vi "NortekCommander.vi"(4 "error in (no error)":errorcluster) -> ()   [LabVIEW 2015]
uses:
  Globals/NortekInstruction.vi
panel:
  out "number":u32
  in  "Stop_Rec":bool
  in  "Start_Rec":bool
  in  "MesureOne":bool
  in  "nom":bool
  out "error out":errorcluster
  out "data out":string
  in  "Date ?":bool
  out "iteration":i32
  in  "Server Closed":string="The server VI closed the connection."
  in  "Stop":bool
  # "Nortek Commander"
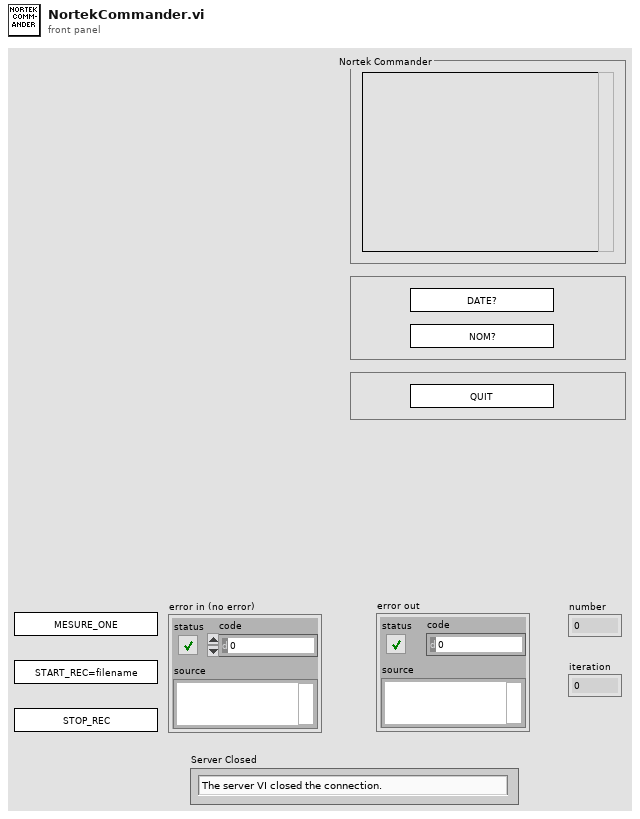
[diagram p1: front panel]
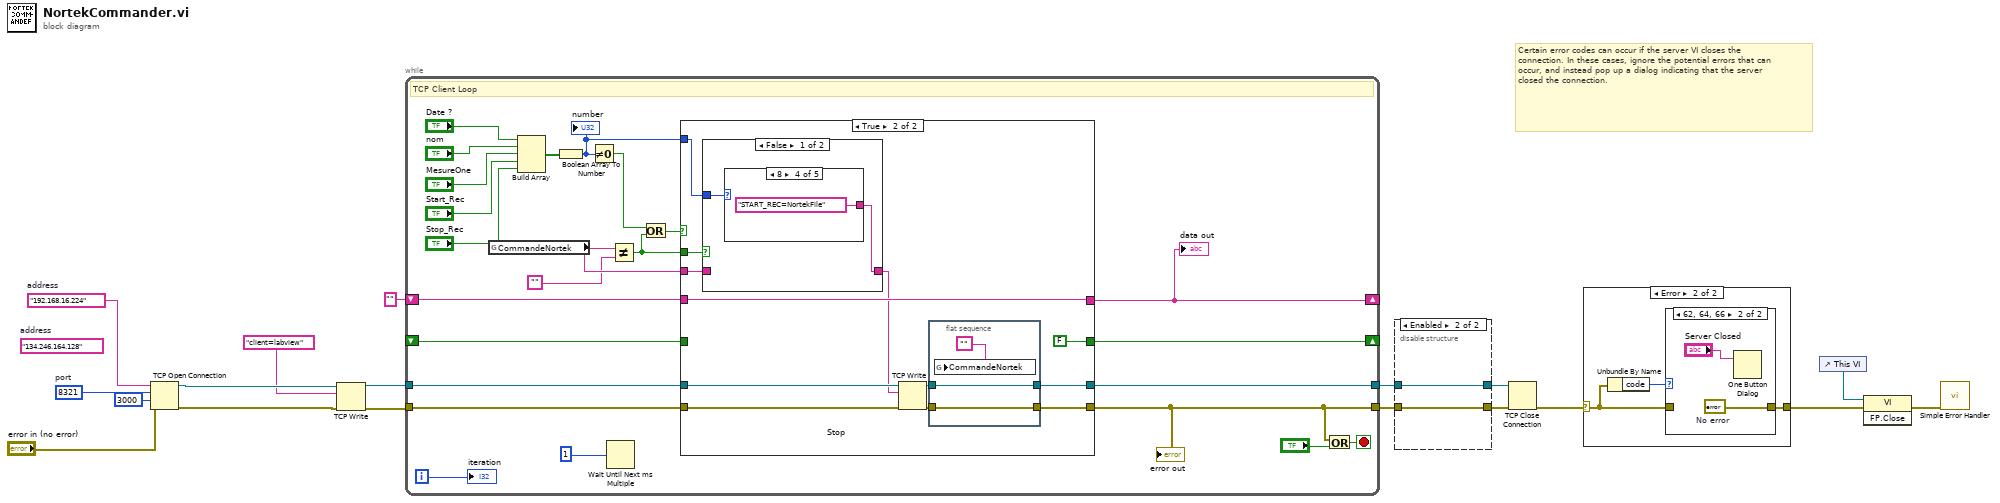
[diagram p0: block diagram]
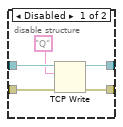
[diagram p2: hidden frame]
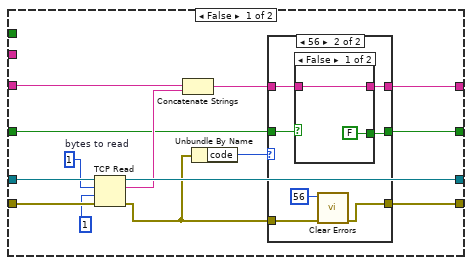
[diagram p5: hidden frame]
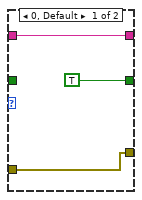
[diagram p6: hidden frame]
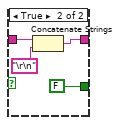
[diagram p7: hidden frame]
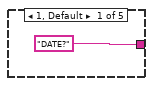
[diagram p8: hidden frame]
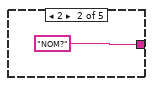
[diagram p9: hidden frame]
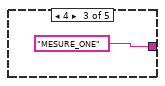
[diagram p10: hidden frame]
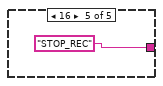
[diagram p11: hidden frame]
diagram:
  w5 = "192.168.16.224"  # address
  w13 = u16 8321  # port
  (unwired) "134.246.164.128"  # address
  # "Certain error codes can occur if the server VI closes the connection. In these cases, ignore the potential errors that can occur, and instead pop up a dialog indicating that the server closed the connection."
  n1 = TCP Open Connection(address=w5, remote port or service name=w13, timeout ms (60000)=3000, error in (no error)="error in (no error)") -> (connection ID=w7:refnum<k5>, error out=w10:errorcluster)  [unwired: 1 in]
  n2 = TCP Write(connection ID=w7, data in="client=labview", error in (no error)=w10) -> (connection ID out=w8:refnum<k5>, error out=w9:errorcluster)  [unwired: 2 out]
  n3 = while {
    tunnel: w9 -> [w39]
    tunnel: w8 -> [w38]
    tunnel: [w37] -> w17
    tunnel: [w34] -> w15
    shift-right: [w35] -> _
    shift-left: "" -> [w36]
    shift-right: [w20] -> _
    shift-left: _ -> [w19]
    i -> [w40]
    stop <- w41 stop-if-true
    # "TCP Client Loop"
    n4 = global read "NortekInstruction.vi" "CommandeNortek"() -> (w23:string)
    n5 = Build Array("Date ?", "nom", "MesureOne", "Start_Rec", "Stop_Rec") -> (w27:bool[])
    n6 = Boolean Array To Number(Boolean array=w27) -> (number=w21:u32)
    "number" <- w21
    n7 = Not Equal To 0?(x=w21) -> (x != 0?=w26:bool)
    n8 = Wait Until Next ms Multiple(millisecond multiple=u32 1) -> ()  [unwired: 1 out]
    n9 = Not Equal?(x=w23, y="") -> (x != y?=w24:bool)
    n10 = Or(x=w26, y=w24) -> (x .or. y?=w25:bool)
    n11 = case shown="True" w25 {
      tunnel: w39 -> [w56 w79]
      tunnel: w38 -> [w55 w78]
      tunnel: [w54 w75] -> w37
      tunnel: w36 -> [w53 w77]
      tunnel: [w43 w77] -> w35
      tunnel: [w52 w80] -> w34
      tunnel: w24 -> [_ w84]
      tunnel: w23 -> [_ w83]
      tunnel: w21 -> [_ w82]
      tunnel: [w46 FALSE] -> w20
      tunnel: w19 -> [w45 _]
      frame False {
        w50 = 1  # bytes to read
        n12 = TCP Read(connection ID=w55, bytes to read=w50, error in (no error)=w56, 9:1 ("timeout ms (25000)")) -> (connection ID out=w54:refnum<k5>, data out=w49:string, error out=w48:errorcluster)  [unwired: 1 in]
        n13 = Concatenate Strings(w53, w49) -> (w44:string)
        n14 = Unbundle By Name(w48) -> ("code"=w47:i32)
        n15 = case shown="56" w47 {
          tunnel: [w59 w66] -> w52
          tunnel: w48 -> [w59 w64]
          tunnel: [TRUE w61] -> w46
          tunnel: w45 -> [_ w63]
          tunnel: [w57 w60] -> w43
          tunnel: w44 -> [w57 w62]
          frame 0, Default {
          }
          frame 56 {
            n16 = case shown="False" w63 {
              tunnel: w62 -> [w68 w71]
              tunnel: [FALSE FALSE] -> w61
              tunnel: [w68 w69] -> w60
              frame False {
              }
              frame True {
                n17 = Concatenate Strings(w71, "\r\n") -> (w69:string)
              }
            }
            n18 = call <vilib>:"Clear Errors.vi"("error in (no error)"=w64, "specific error code to clear (0: all)"=56) -> ("error out"=w66:errorcluster)  [unwired: 4 in, 1 out]
          }
        }
      }
      frame True {
        n19 = case shown="False" w84 {
          tunnel: w83 -> [_ w95]
          tunnel: w82 -> [w89 _]
          tunnel: [w88 w95] -> w76
          frame False {
            n20 = case shown="8" w89 {
              tunnel: ["DATE?" "NOM?" "MESURE_ONE" "START_REC=NortekFile" "STOP_REC"] -> w88
              frame 1, Default {
              }
              frame 2 {
              }
              frame 4 {
              }
              frame 8 {
              }
              frame 16 {
              }
            }
          }
          frame True {
          }
        }
        n21 = TCP Write(connection ID=w78, data in=w76, error in (no error)=w79) -> (connection ID out=w74:refnum<k5>, error out=w81:errorcluster)  [unwired: 2 out]
        n22 = flat-sequence {
          tunnel: [w87] -> w80
          tunnel: w81 -> [w87]
          tunnel: [w85] -> w75
          tunnel: w74 -> [w85]
          frame #0 {
            n23 = global write "NortekInstruction.vi" "CommandeNortek"("") -> ()
          }
        }
      }
    }
    "error out" <- w34
    "data out" <- w35
    n24 = Or(x=w34, y="Stop") -> (x .or. y?=w41:bool)
    "iteration" <- w40
  }
  n25 = disable-structure shown="Enabled" {
    disable-tunnel: [w100 w102] -> w18
    disable-tunnel: w17 -> [w99 w102]
    disable-tunnel: [w98 w101] -> w16
    disable-tunnel: w15 -> [w97 w101]
    frame Disabled {
      n26 = TCP Write(connection ID=w99, data in="Q", error in (no error)=w97) -> (connection ID out=w100:refnum<k5>, error out=w98:errorcluster)  [unwired: 2 out]
    }
    frame Enabled {
    }
  }
  n27 = TCP Close Connection(connection ID=w18, error in (no error)=w16) -> (error out=w14:errorcluster)  [unwired: 1 in, 1 out]
  n28 = case shown="Error" w14 {
    selector: w14 -> [w103 w105]
    tunnel: [w103 w104] -> w3
    frame No Error {
    }
    frame Error {
      n29 = Unbundle By Name(w105) -> ("code"=w106:i32)
      n30 = case shown="62, 64, 66" w106 {
        tunnel: w105 -> [w107 _]
        tunnel: [w107 w109] -> w104
        frame Default {
        }
        frame 62, 64, 66 {
          w109 = errorcluster {"status"=FALSE, "code"=0, "source"=""}  # No error
          n31 = One Button Dialog(message="Server Closed") -> ()  [unwired: 1 in, 1 out]
        }
      }
    }
  }
  n32 = control-ref of="This VI"() -> (w4:refnum<vi>)
  n33 = invoke class="VI" method="FP.Close"(reference=w4, error in=w3) -> (error out=w2:errorcluster)  [unwired: 1 in, 2 out]
  n34 = call <vilib>:"Simple Error Handler.vi"("error in (no error)"=w2) -> ()  [unwired: 4 in, 5 out]
